vi "ep_Caculate Time Position.vi"(0 "reference signal":dbl[](array[numeric]), 2 "reset? (F)":bool, 5 "parameters":T1, 9 "system info in":refnum<class "EP System Info.lvclass">, 11 "error in (no error)":errorcluster) -> (4 "sampling rate [Hz]":dbl format="%.6f", 6 "time position":dbl[](array[numeric]), 10 "system info out":refnum<class "EP System Info.lvclass">, 15 "error out":errorcluster)   [LabVIEW 2012, in "NI_EP_Resample_Host.lvlib"]
uses:
  <vilib>/addons/Electrical Power/PQ/Resampling/NI_EP_Resample_Host.lvlib
  <vilib>/addons/Electrical Power/PQ/Common/Classes/System Info/EP System Info.lvclass
  <vilib>/addons/Electrical Power/PQ/Resampling/Desktop/subVIs/ep_Parameters.ctl
  <vilib>/Analysis/baseanly.llb/Mean (DBL).vi
  <vilib>/Analysis/1siggen.llb/Ramp Pattern by Samples.vi
  <vilib>/Analysis/NI_AALBase.lvlib
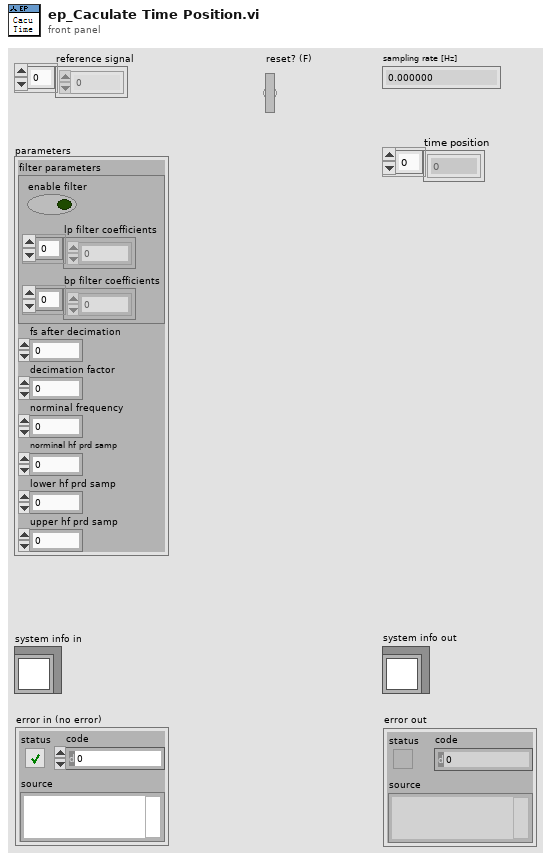
[diagram p1: front panel]
types:
  T1 = typedef "NI_EP_Resample_Host.lvlib/ep_Parameters.ctl" = cluster{"filter parameters":cluster{"enable filter":bool, "lp filter coefficients":dbl[], "bp filter coefficients":dbl[]}, "fs after decimation":dbl, "decimation factor":i32, "norminal frequency":dbl, "norminal hf prd samp":dbl, "lower hf prd samp":i32, "upper hf prd samp":i32}
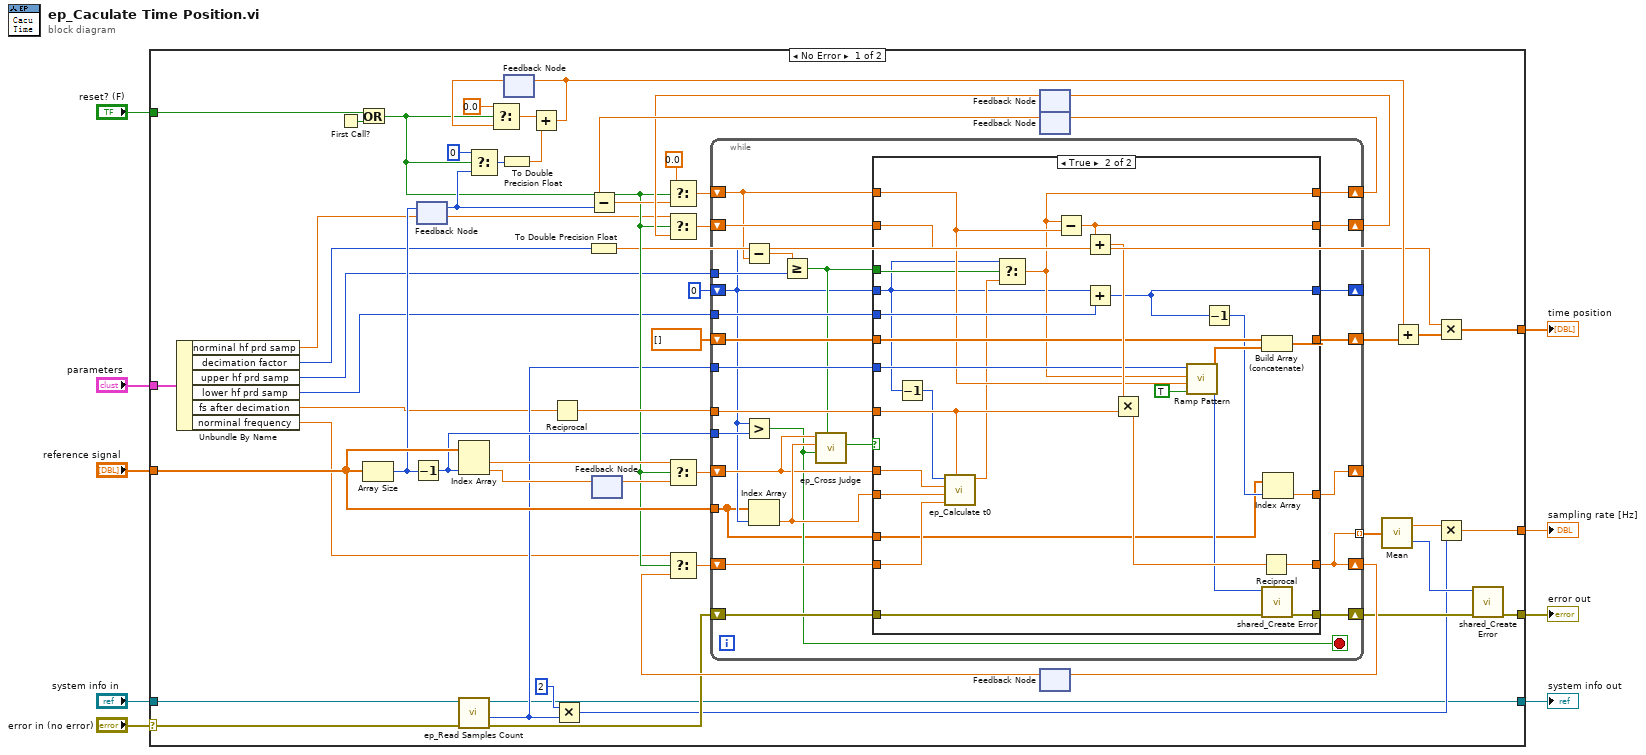
[diagram p0: block diagram]
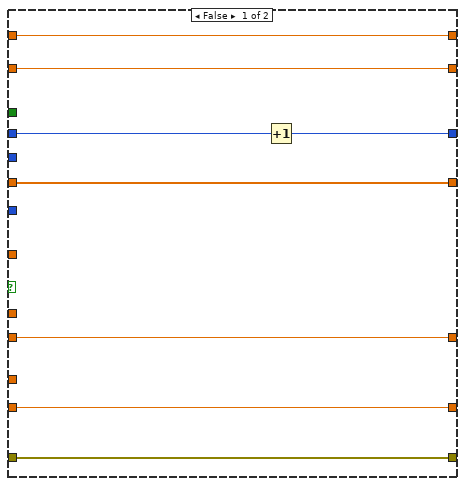
[diagram p2: hidden frame]
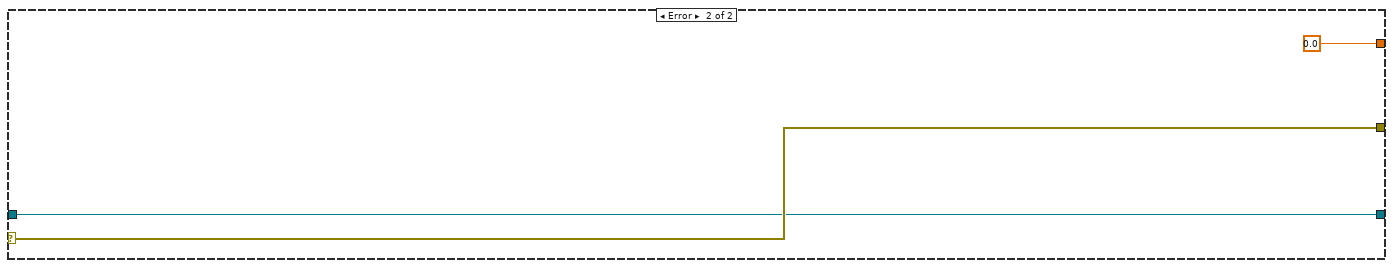
[diagram p3: hidden frame]
diagram:
  n1 = case shown="No Error" "error in (no error)" {
    selector: "error in (no error)" -> [w23 w129]
    tunnel: "reference signal" -> [w62 _]
    tunnel: [w64 w129] -> w8
    tunnel: "reset? (F)" -> [w65 _]
    tunnel: [w63 _] -> w3
    tunnel: [w10 0.0 ("mean")] -> w6
    tunnel: [w18 w127] -> w5
    tunnel: "system info in" -> [w24 w127]
    tunnel: "parameters" -> [w11 _]
    frame No Error {
      n2 = Unbundle By Name(w11) -> ("norminal hf prd samp"=w17:dbl, "decimation factor"=w16:i32, "upper hf prd samp"=w15:i32, "lower hf prd samp"=w14:i32, "fs after decimation"=w13:dbl, "norminal frequency"=w12:dbl)
      n3 = First Call?() -> (First Call?: T/F=w51:bool)
      n4 = Or(x=w65, y=w51) -> (x .or. y?=w28:bool)
      n5 = Array Size(array=w62) -> (size(s)=w33:i32)
      n6 = Decrement(x=w33) -> (x-1=w25:i32)
      n7 = feedback #1() -> (w43:i32)  [unwired: 1 in]
      n8 = feedback-in #1(w33) -> ()
      n9 = Index Array(array=w62, index #2=w25) -> (element #1=w56:dbl, element #2=w59:dbl)  [unwired: 1 in]
      n10 = call <vilib>:"ep_Read Samples Count.vi"("error in (no error)"=w23, "system info in"=w24) -> ("error out"=w22:errorcluster, "half-cycle (samples)"=w21:i32, "system info out"=w18:refnum<class "EP System Info.lvclass">)  [unwired: 5 in, 2 out]
      n11 = Select(t=0, s=w28, f=w43) -> (s? t:f=w44:i32)
      n12 = To Double Precision Float(number=w44) -> (double precision float=w40:dbl)
      n13 = feedback #2() -> (w37:dbl)  [unwired: 1 in]
      n14 = Select(t=0.0, s=w28, f=w37) -> (s? t:f=w39:dbl)
      n15 = Add(x=w39, y=w40) -> (x+y=w35:dbl)
      n16 = feedback-in #2(w35) -> ()
      n17 = Reciprocal(x=w13) -> (1/x=w41:dbl)
      n18 = Multiply(x=2 ("y"), y=w21) -> (x*y=w19:i32)
      n19 = To Double Precision Float(number=w16) -> (double precision float=w26:dbl)
      n20 = feedback #3() -> (w55:dbl)  [unwired: 1 in]
      n21 = feedback-in #3(w59) -> ()
      n22 = Select(t=w56, s=w28, f=w55) -> (s? t:f=w54:dbl)
      n23 = feedback #4() -> (w53:dbl)  [unwired: 1 in]
      n24 = Select(t=w17, s=w28, f=w53) -> (s? t:f=w52:dbl)
      n25 = feedback #5() -> (w60:dbl)  [unwired: 1 in]
      n26 = Subtract(x=w60, y=w43) -> (x-y=w32:dbl)
      n27 = Select(t=0.0, s=w28, f=w32) -> (s? t:f=w50:dbl)
      n28 = feedback #6() -> (w48:dbl)  [unwired: 1 in]
      n29 = Select(t=w12, s=w28, f=w48) -> (s? t:f=w47:dbl)
      n30 = while {
        shift-right: [w67] -> _
        shift-left: w54 -> [w73]
        tunnel: w62 -> [w66]
        shift-right: [w90] -> _
        shift-left: 0 -> [w68]
        shift-right: [w83] -> w58
        shift-left: w50 -> [w69]
        tunnel: w41 -> [w89]
        shift-right: [w88] -> w57
        shift-left: w52 -> [w87]
        shift-right: [w76] -> w46
        shift-left: w47 -> [w86]
        shift-right: [w82] -> w36
        shift-left: dbl[] [] -> [w81]
        tunnel: [w76] -> w29 mode=indexing
        tunnel: w14 -> [w80]
        tunnel: w21 -> [w79]
        tunnel: w25 -> [w72]
        tunnel: w15 -> [w70]
        shift-right: [w77] -> w31
        shift-left: w22 -> [w78]
        stop <- w71 stop-if-true
        n31 = Subtract(x=w68, y=w69) -> (x-y=w75:dbl)
        n32 = Greater?(x=w68, y=w72) -> (0:w71:bool)
        n33 = Index Array(array=w66, index=w68) -> (element=w85:dbl)
        n34 = Greater Or Equal?(x=w75, y=w70) -> (x >= y?=w74:bool)
        n35 = call <vilib>:"ep_Cross Judge.vi"("over threshold?"=w74, "over index?"=w71, "y2"=w85, "y1"=w73) -> ("cross"=w84:bool)  [unwired: 7 in]
        n36 = case shown="True" w84 {
          tunnel: w68 -> [w98 w103]
          tunnel: [w97 w101] -> w90
          tunnel: w73 -> [_ w121]
          tunnel: w85 -> [w91 w122]
          tunnel: [w96 w106] -> w83
          tunnel: w69 -> [w96 w107]
          tunnel: w89 -> [_ w120]
          tunnel: [w95 w126] -> w88
          tunnel: w87 -> [w95 w125]
          tunnel: [w94 w123] -> w76
          tunnel: w86 -> [w94 w116]
          tunnel: [w93 w115] -> w82
          tunnel: w81 -> [w93 w109]
          tunnel: w80 -> [_ w117]
          tunnel: w79 -> [_ w108]
          tunnel: w78 -> [w92 w112]
          tunnel: [w92 w111] -> w77
          tunnel: w74 -> [_ w104]
          tunnel: [w91 w102] -> w67
          tunnel: w66 -> [_ w99]
          frame False {
            n37 = Increment(x=w98) -> (x+1=w97:i32)
          }
          frame True {
            n38 = Decrement(x=w103) -> (x-1=w118:i32)
            n39 = call <vilib>:"ep_Calculate t0.vi"("dt"=w120, "freq"=w116, "y2"=w122, "y1"=w121, "t1"=w118) -> ("t0"=w105:dbl)  [unwired: 6 in]
            n40 = Select(t=w103, s=w104, f=w105) -> (s? t:f=w106:dbl)
            n41 = Subtract(x=w106, y=w107) -> (x-y=w126:dbl)
            n42 = Add(x=w126, y=w125) -> (x+y=w119:dbl)
            n43 = Add(x=w103, y=w117) -> (x+y=w101:i32)
            n44 = Multiply(x=w119, y=w120) -> (x*y=w124:dbl)
            n45 = call-poly <vilib>:"Ramp Pattern.vi"("exclude end?"=TRUE, "start"=w107, "end"=w106, "samples"=w108) -> ("error"=w113:i32, "Ramp Pattern"=w110:dbl[])  [unwired: 6 in]
            n46 = Decrement(x=w101) -> (x-1=w100:i32)
            n47 = Reciprocal(x=w124) -> (1/x=w123:dbl)
            n48 = Build Array (concatenate)(w109, w110) -> (w115:dbl[])
            n49 = call <vilib>:"shared_Create Error.vi"("error in (no error)"=w112, "error code (0)"=w113) -> ("error out"=w111:errorcluster)  [unwired: 9 in]
            n50 = Index Array(array=w99, index=w100) -> (element=w102:dbl)
          }
        }
      }
      n51 = feedback-in #4(w57) -> ()
      n52 = feedback-in #5(w58) -> ()
      n53 = feedback-in #6(w46) -> ()
      n54 = call-poly <vilib>:"Mean.vi"("X"=w29) -> ("mean"=w27:dbl, "error"=w30:i32)
      n55 = Add(x=w35, y=w36) -> (x+y=w34:dbl[])
      n56 = Multiply(x=w26, y=w34) -> (x*y=w63:dbl[])
      n57 = Multiply(x=w27, y=w19) -> (x*y=w10:dbl)
      n58 = call <vilib>:"shared_Create Error.vi"("error in (no error)"=w31, "error code (0)"=w30) -> ("error out"=w64:errorcluster)  [unwired: 9 in]
    }
    frame Error {
    }
  }
  "error out" <- w8
  "sampling rate [Hz]" <- w6
  "system info out" <- w5
  "time position" <- w3
